vi "read file from 5071C.vi"(8 "error in (no error)":errorcluster, 10 "状态名":string, 11 "VISA resource name":refnum<visa-resource-name>="E5071C") -> (0 "error out":errorcluster={"status"=FALSE, "code"=1073676294, "source"="VISA Read in Untitled 2"}, 3 "VISA resource name out":refnum<visa-resource-name>="E5071C")   [LabVIEW 2011]
uses:
  Agilent ENA Series/Agilent ENA Series.lvlib
panel:
  out "read buffer":string="#6043969"
  out "Return Count":i32=43970
  out "Data Block ()":string
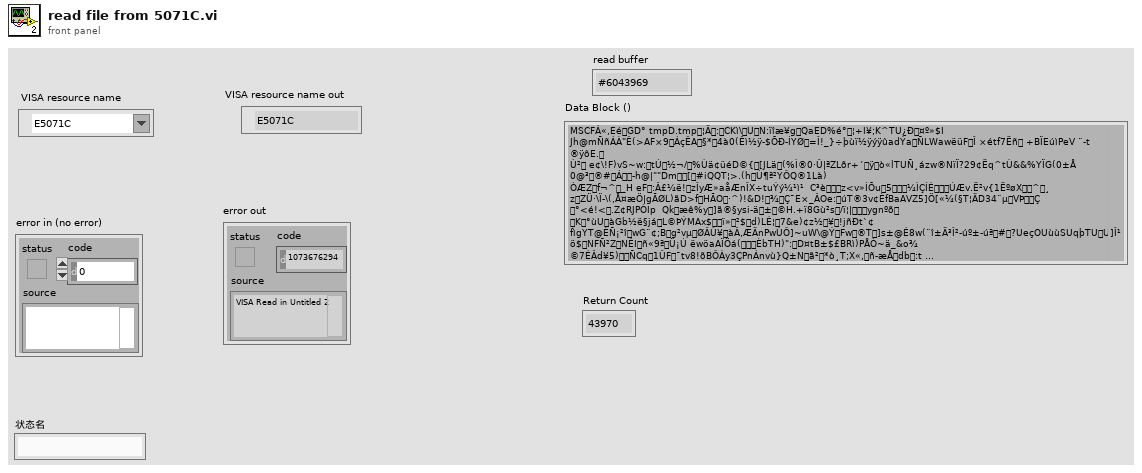
[diagram p1: front panel]
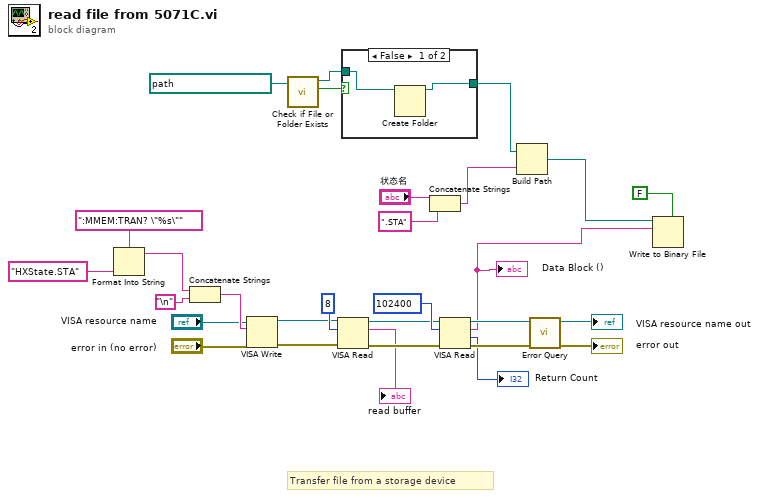
[diagram p0: block diagram]
diagram:
  # "Transfer file from a storage device"
  n1 = Format Into String(format string=":MMEM:TRAN? \"%s\"", "HXState.STA" ("File Name ()")) -> (resulting string=w22:string)  [unwired: 2 in, 1 out]
  n2 = Concatenate Strings(w22, "\n") -> (w24:string)
  n3 = VISA Write(VISA resource name="VISA resource name", write buffer=w24, error in (no error)="error in (no error)") -> (VISA resource name out=w15:refnum<visa-resource-name>, error out=w13:errorcluster)  [unwired: 1 out]
  n4 = call <vilib>:"Check if File or Folder Exists.vi"("path"=path "D:/E5071C校准状态" ("本机文件")) -> ("file or folder exists?"=w3:bool, "dup path"=w2:path)  [unwired: 8 in, 1 out]
  n5 = VISA Read(VISA resource name=w15, byte count=u32 8, error in (no error)=w13) -> (VISA resource name out=w14:refnum<visa-resource-name>, read buffer=→"read buffer":string, error out=w12:errorcluster)  [unwired: 1 out]
  n6 = case shown="False" w3 {
    tunnel: w2 -> [w30 w32]
    tunnel: [w31 w32] -> w1
    frame False {
      n7 = Create Folder(path (use dialog)=w30) -> (created path=w31:path)  [unwired: 2 in, 2 out]
    }
    frame True {
    }
  }
  n8 = Concatenate Strings("状态名", ".STA" ("string")) -> (w6:string)
  n9 = VISA Read(VISA resource name=w14, byte count=u32 102400, error in (no error)=w12) -> (VISA resource name out=w19:refnum<visa-resource-name>, read buffer=w10:string, return count=→"Return Count":u32, error out=w18:errorcluster)
  "Data Block ()" <- w10
  n10 = Build Path(base path=w1, name or relative path=w6) -> (appended path=w8:path)
  n11 = call "Error Query.vi"("error in (no error)"=w18, "VISA resource name"=w19) -> ("error out"=→"error out":errorcluster, "VISA resource name out"=→"VISA resource name out":refnum<visa-resource-name>)  [unwired: 6 in, 2 out]
  n12 = Write to Binary File(file (use dialog)=w8, data=w10, 5:FALSE ("prepend array or string size? (T)")) -> ()  [unwired: 3 in, 3 out]
